vi "Write Channel.vi"(8 "error in (no error)":errorcluster, 10 "Channel":dbl, 11 "Read DMM in":refnum<class "Read DMM.lvclass">) -> (0 "error out":errorcluster, 3 "Read DMM out":refnum<class "Read DMM.lvclass">)   [LabVIEW 2020, in "Read DMM.lvclass"]
uses:
  Read DMM.lvclass
  Read DMM.lvclass/Read DMM.ctl
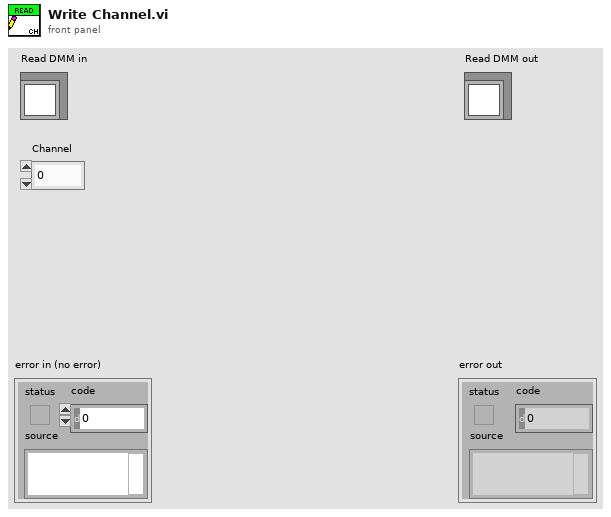
[diagram p1: front panel]
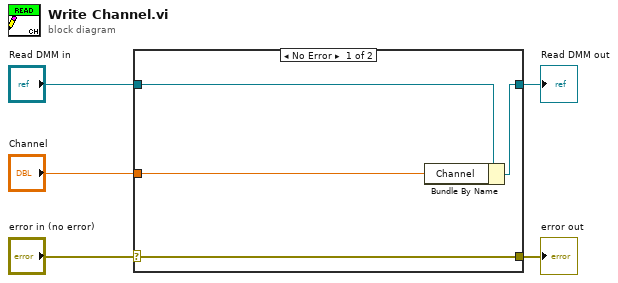
[diagram p0: block diagram]
diagram:
  n1 = case shown="No Error" "error in (no error)" {
    selector: "error in (no error)" -> [w9 w10]
    tunnel: [w9 w10] -> w4
    tunnel: [w7 w11] -> w2
    tunnel: "Read DMM in" -> [w8 w11]
    tunnel: "Channel" -> [w6 _]
    frame No Error {
      n2 = Bundle By Name(cluster=w8, "Channel"=w6) -> (w7:refnum<class "Read DMM.lvclass">)
    }
    frame Error {
    }
  }
  "error out" <- w4
  "Read DMM out" <- w2
